vi "Read Single.vi"(8 "error in (no error)":errorcluster, 10 "Timeout (msec)":i32=-1, 11 "Session Handle":refnum<k15>) -> (0 "error out":errorcluster, 2 "Measurement":dbl format="%.5f", 3 "instrument handle out":refnum<k15> caption="Session Handle Out")   [LabVIEW 2026, in "PXI4072.lvlib"]
uses:
  PXI4072.lvlib
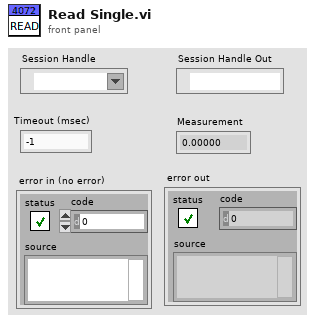
[diagram p1: front panel]
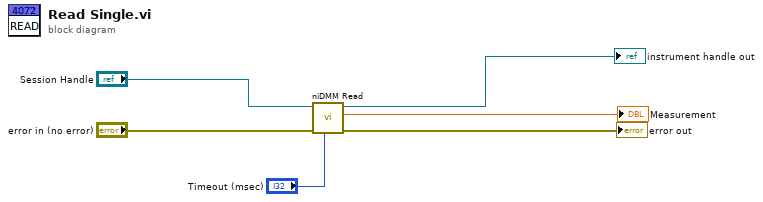
[diagram p0: block diagram]
diagram:
  n1 = call <instrlib>:"niDMM Read.vi"("Maximum Time (msec)"="Timeout (msec)", "error in (no error)"="error in (no error)", "instrument handle"="Session Handle") -> ("error out"=→"error out":errorcluster, "Measurement"=→"Measurement":dbl, "instrument handle out"=→"instrument handle out":refnum<k15>)  [unwired: 6 in]
